vi "Init from Existing Queue.vi"(10 "Priority Queue":refnum<class "Message Priority Queue.lvclass">) -> (3 "Message Enqueuer":refnum<class "Message Enqueuer.lvclass">)   [LabVIEW 2020, in "Actor Framework.lvlib" / "Message Enqueuer.lvclass"]
uses:
  Message Enqueuer.lvclass
  Message Priority Queue/Message Priority Queue.lvclass
  Message Enqueuer.lvclass/Message Enqueuer.ctl
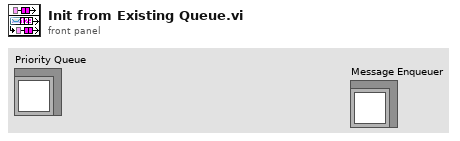
[diagram p1: front panel]
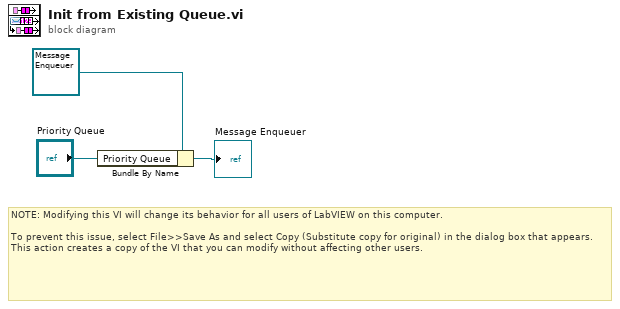
[diagram p0: block diagram]
diagram:
  # "NOTE: Modifying this VI will change its behavior for all users of LabVIEW on this computer.\n\nTo prevent this issue, select File>>Save As and select Copy (Substitute copy for original) in the dialog box that appears. This action creates a copy of the VI that you can modify without affecting other users."
  n1 = Bundle By Name(cluster=refnum<class "Message Enqueuer.lvclass"> refnum ("Actor Framework.lvlib:Message Enqueuer.lvclass"), "Priority Queue"="Priority Queue") -> (→"Message Enqueuer":refnum<class "Message Enqueuer.lvclass">)
